vi "UTF-8 Path Probe.vi"(1 "UTF-8 Path":refnum<class "UTF-8 Path.lvclass">) -> (0 "Boolean":bool)   [LabVIEW 2020, in "G-Unicode.lvlib" / "UTF-8 Path.lvclass"]
uses:
  UTF-8 Path.lvclass
  G-Unicode.lvlib
  Unicode/Controls/String Encoding.ctl
panel:
  out "Unicode":string
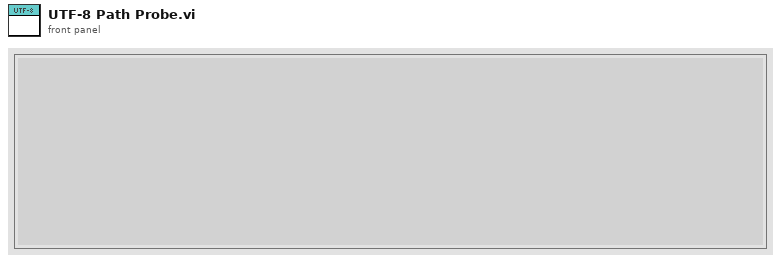
[diagram p1: front panel]
types:
  T1 = typedef "G-Unicode.lvlib/String Encoding.ctl" = enum16{"ANSI", "UTF-8", "UTF-16LE", "UTF-16BE", "Unknown"}
  T2 = typedef "G-Unicode.lvlib/Encoded UTF-8 Path.ctl" = path
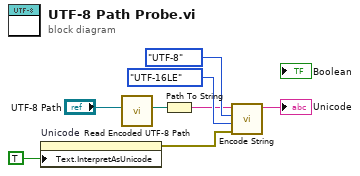
[diagram p0: block diagram]
diagram:
  n1 = property on="Unicode" class="Str"("Text.InterpretAsUnicode"=TRUE ("Force Unicode Text")) -> (error out=w6:errorcluster)  [unwired: 2 in, 1 out]
  n2 = call "Read Encoded UTF-8 Path.vi"("UTF-8 Path"="UTF-8 Path") -> ("Encoded UTF-8 Path"=w3:T2)  [unwired: 10 in]
  n3 = Path To String(path=w3) -> (string=w1:string)
  n4 = call "Encode String.vi"("error in"=w6, "Output Encoding (UTF-16LE)"=String_Encoding."UTF-16LE" ("Output Encoding (UTF-8)"), "Input Encoding (ANSI)"=String_Encoding."UTF-8", "String in"=w1) -> ("String out"=→"Unicode":string)  [unwired: 6 in, 1 out]
